vi "QA.vi"(8 "ERRIN":errorcluster caption="entrée d'erreur (pas d'erreur)") -> (0 "ERROUT":errorcluster caption="sortie d'erreur", 2 "DATAOUT":string)   [LabVIEW 2020]
uses:
  <vilib>/Instr/_visa.llb/VISA Configure Serial Port (Instr).vi
panel:
  in  "buffer d'écriture":string
  # "<\\B20\\BE:(A\\CC\\A9:P\\D2\\C5SS\\C9\\CFN\\A0HAU\\D4\\C5\\8D\\n"
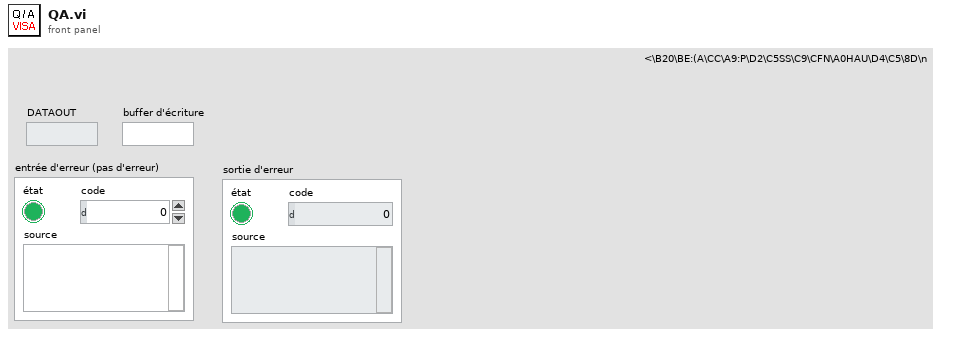
[diagram p1: front panel]
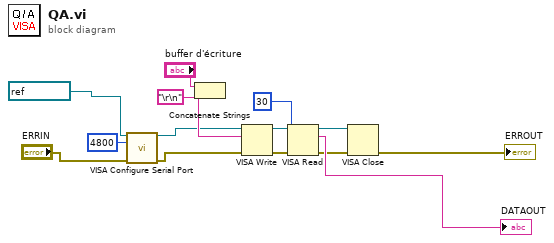
[diagram p0: block diagram]
diagram:
  n1 = call-poly "VISA Configure Serial Port"("VISA resource name"=refnum<visa-resource-name> "COM8" ("Refnum VISA en sortie"), "baud rate (9600)"=u32 4800, "error in (no error)"="ERRIN") -> ("VISA resource name out"=w1:refnum<visa-resource-name>, "error out"=w4:errorcluster)  [unwired: 11 in]
  n2 = Concatenate Strings("buffer d'écriture", "\r\n") -> (w6:string)
  n3 = VISA Write(VISA resource name=w1, write buffer=w6, error in (no error)=w4) -> (VISA resource name out=w9:refnum<visa-resource-name>, error out=w11:errorcluster)  [unwired: 1 out]
  n4 = VISA Read(VISA resource name=w9, byte count=u32 30 ("nombre d'octets"), error in (no error)=w11) -> (VISA resource name out=w12:refnum<visa-resource-name>, read buffer=→"DATAOUT":string, error out=w13:errorcluster)  [unwired: 1 out]
  n5 = VISA Close(VISA resource name=w12, error in (no error)=w13) -> (error out=→"ERROUT":errorcluster)
